vi "FRC myRIO v1.0 Read I2C.vi"(4 "Keep Bus Busy":bool, 6 "Slave Address (7-bit)":u8, 7 "Timeout ms (5)":i32=5, 8 "Error In (No Error)":errorcluster, 9 "Bytes to Read":u32) -> (0 "error out":errorcluster, 2 "Data Read":u8[](array[numeric]))   [LabVIEW 2017]
uses:
  <vilib>/rvi/errors/niLvFpgaAdjustHostInterfaceError.vi
  <vilib>/Rock Robotics/SystemInterfaces/System/FPGA_SystemFRC FPGA Ref.ctl
  <vilib>/rvi/interface/nirviReadWriteControl/nirviReadWriteControl.xnode
  NiFpgaLv.dll
  <vilib>/rvi/interface/Simulation/niFpgaSimulationCallBeginRW.vi
panel:
  # "This VI writes an array of data to the SPI Data Out register (SPIn.SPDO) and reads an array of data from the SPI Data In register (SPIn.SPDI) for a particular SPI channel (n). The data is written/read one value at a time. Please see Block Diagram for details."
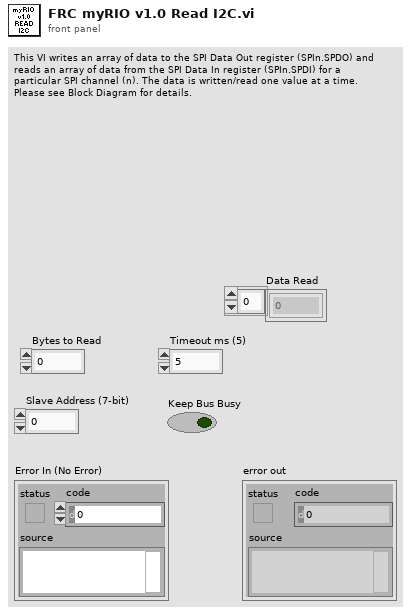
[diagram p1: front panel]
types:
  T1 = typedef "FPGA_SystemFRC FPGA Ref.ctl" = refnum<k20>
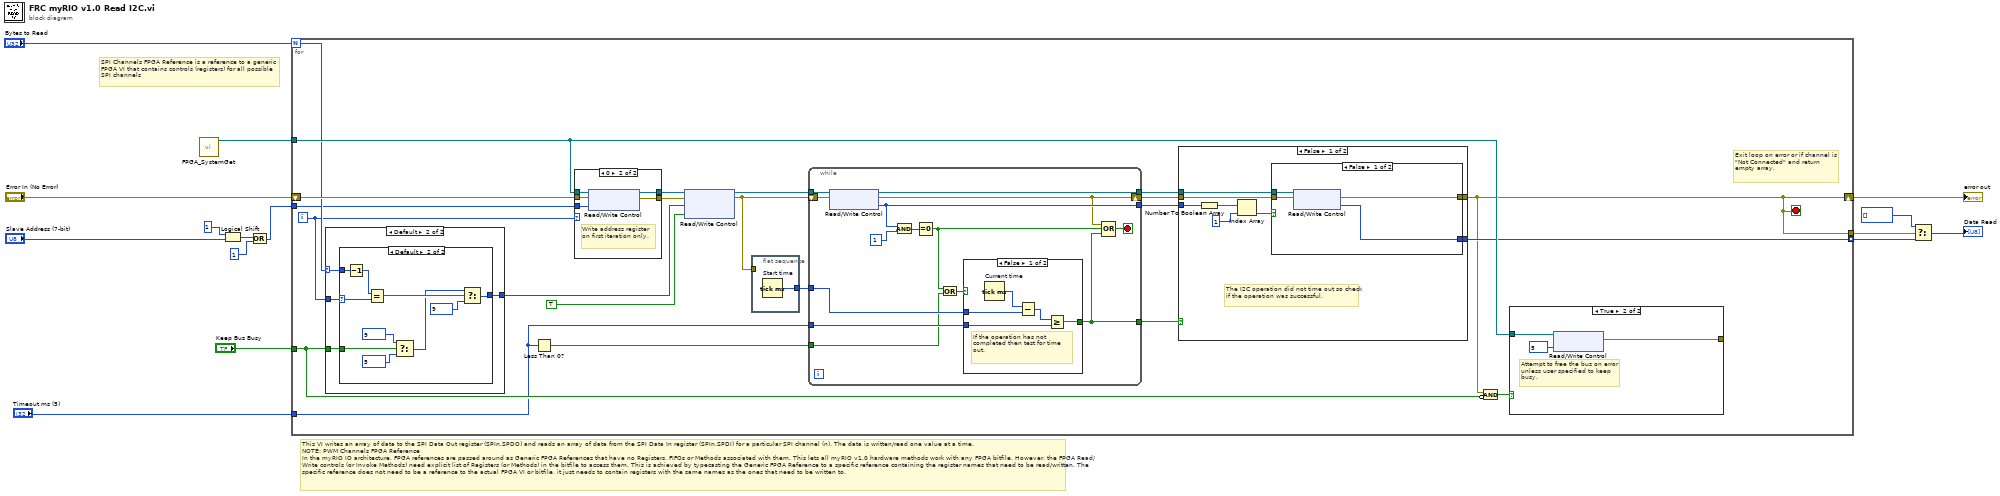
[diagram p0: block diagram]
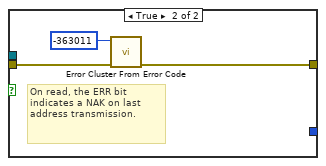
[diagram p2: hidden frame]
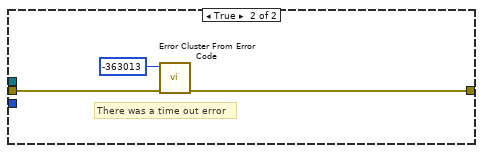
[diagram p3: hidden frame]
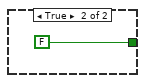
[diagram p6: hidden frame]
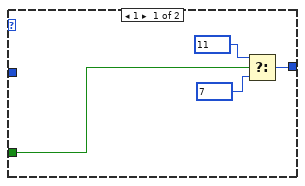
[diagram p7: hidden frame]
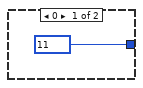
[diagram p8: hidden frame]
diagram:
  # "This VI writes an array of data to the SPI Data Out register (SPIn.SPDO) and reads an array of data from the SPI Data In register (SPIn.SPDI) for a particular SPI channel (n). The data is written/read one value at a time.\nNOTE: PWM Channels FPGA Reference\nIn the myRIO IO architecture, FPGA references are passed around as Generic FPGA References that have no Registers, FIFOs or Methods associated with them. This lets all myRIO v1.0 hardware methods work with any FPGA bitfile. However, the FPGA Read/Write controls (or Invoke Methods) need explicit list of Registers (or Methods) in the bitfile to access them. This is achieved by typecasting the Generic FPGA Reference to a specific reference containing the register names that need to be read/written. The specific reference does not need to be a reference to the actual FPGA VI or bitfile, it just needs to contain registers with the same names as the ones that need to be written to."
  # "SPI Channels FPGA Reference is a reference to a generic FPGA VI that contains controls (registers) for all possible SPI channels"
  n1 = call <vilib>:"FPGA_SystemGet.vi"() -> ("FRC FPGA Ref"=w1:T1)  [unwired: 11 in]
  n2 = Logical Shift(y=i8 1, x="Slave Address (7-bit)") -> (x << y=w13:u8)
  n3 = Or(x=w13, y=u8 1) -> (x .or. y?=w3:u8)
  n4 = for {
    N: "Bytes to Read" -> [w33]
    shift-right: [w16] -> w7
    shift-left: "Error In (No Error)" -> [w37]
    tunnel: w1 -> [w36]
    tunnel: [w32] -> w5 mode=indexing
    tunnel: [w16] -> w6
    tunnel: "Keep Bus Busy" -> [w29]
    tunnel: w3 -> [w31]
    tunnel: "Timeout ms (5)" -> [w28]
    i -> [w30]
    stop <- w16 stop-if-true
    # "Exit loop on error or if channel is \"Not Connected\" and return empty array."
    n5 = case shown="Default" w33 {
      selector: w33 -> [_ w92]
      tunnel: [w90 w93] -> w34
      tunnel: w30 -> [_ w94]
      tunnel: w29 -> [w88 w91]
      frame 1 {
        n6 = Select(t=u8 11 ("y"), s=w88, f=u8 7 ("y")) -> (s? t:f=w90:u8)
      }
      frame Default {
        n7 = case shown="Default" w94 {
          selector: w94 -> [_ w103]
          tunnel: [u8 11 ("y") w101] -> w93
          tunnel: w92 -> [_ w105]
          tunnel: w91 -> [_ w98]
          frame 0 {
          }
          frame Default {
            n8 = Decrement(x=w105) -> (x-1=w104:i32)
            n9 = Equal?(x=w104, y=w103) -> (x = y?=w102:bool)
            n10 = Select(t=u8 9 ("y"), s=w98, f=u8 5 ("y")) -> (s? t:f=w97:u8)
            n11 = Select(t=w97, s=w102, f=u8 9 ("y")) -> (s? t:f=w101:u8)
          }
        }
      }
    }
    n12 = Less Than 0?(x=w28) -> (x < 0?=w27:bool)
    n13 = case shown="0" w30 {
      tunnel: [w61 w66] -> w22
      tunnel: [w60 w65] -> w21
      tunnel: w36 -> [w61 w64]
      tunnel: w37 -> [w60 w63]
      tunnel: w31 -> [_ w62]
      frame Default {
      }
      frame 0 {
        # "Write address register on first iteration only."
        n14 = xnode "Read/Write Control"("FPGA VI Reference In"=w64, "error in"=w63, "Accel.ADDR"=w62) -> ("FPGA VI Reference Out"=w66:T1, "error out"=w65:errorcluster)
      }
    }
    n15 = xnode "Read/Write Control"("FPGA VI Reference In"=w22, "error in"=w21, "Accel.CNTL"=w34, "Accel.GO"=TRUE ("I2C0.GO")) -> ("FPGA VI Reference Out"=w26:T1, "error out"=w17:errorcluster)
    n16 = flat-sequence {
      tunnel: [w38] -> w19
      tunnel: w17 -> [_]
      frame #0 {
        n17 = Tick Count (ms) "Start time"() -> (millisecond timer value=w38:u32)
      }
    }
    n18 = while {
      tunnel: w26 -> [w79]
      shift-right: [w73] -> w25
      shift-left: w17 -> [w80]
      tunnel: [w75] -> w24
      tunnel: [w74] -> w23
      tunnel: w19 -> [w72]
      tunnel: [w71] -> w18
      tunnel: w28 -> [w70]
      tunnel: w27 -> [w68]
      stop <- w76 stop-if-true
      n19 = xnode "Read/Write Control"("FPGA VI Reference In"=w79, "error in"=w80) -> ("FPGA VI Reference Out"=w74:T1, "error out"=w73:errorcluster, "Accel.STAT"=w75:u8)
      n20 = And(x=w75, y=u8 1) -> (x .and. y?=w77:u8)
      n21 = Equal To 0?(x=w77) -> (x = 0?=w67:bool)
      n22 = Or(x=w67, y=w68) -> (x .or. y?=w69:bool)
      n23 = case shown="False" w69 {
        tunnel: w72 -> [w83 _]
        tunnel: [w82 FALSE] -> w71
        tunnel: w70 -> [w81 _]
        frame False {
          # "If the operation has not completed then test for time out."
          n24 = Tick Count (ms) "Current time"() -> (millisecond timer value=w84:u32)
          n25 = Subtract(x=w84, y=w83) -> (x-y=w85:u32)
          n26 = Greater Or Equal?(x=w85, y=w81) -> (x >= y?=w82:bool)
        }
        frame True {
        }
      }
      n27 = Compound Arithmetic op=OR(w73, w67, w71) -> (w76:bool)
    }
    n28 = case shown="False" w18 {
      tunnel: w25 -> [w46 w55]
      tunnel: w24 -> [w45 _]
      tunnel: [w41 _] -> w32
      tunnel: w23 -> [w40 _]
      tunnel: [w39 w54] -> w16
      frame False {
        # "The I2C operation did not time out so check if the operation was successful."
        n29 = Number To Boolean Array(number=w45) -> (Boolean array=w44:bool[])
        n30 = Index Array(array=w44, index=1) -> (element=w43:bool)
        n31 = case shown="False" w43 {
          tunnel: w46 -> [w48 w51]
          tunnel: [w49 w53] -> w39
          tunnel: [w50 _] -> w41
          tunnel: w40 -> [w47 _]
          frame False {
            n32 = xnode "Read/Write Control"("FPGA VI Reference In"=w47, "error in"=w48) -> ("error out"=w49:errorcluster, "Accel.DATI"=w50:u8)  [unwired: 1 out]
          }
          frame True {
            # "On read, the ERR bit indicates a NAK on last address transmission."
            n33 = call <vilib>:"Error Cluster From Error Code.vi"("error in (no error)"=w51, "error code (0)"=-363011) -> ("error out"=w53:errorcluster)  [unwired: 7 in]
          }
        }
      }
      frame True {
        # "There was a time out error"
        n34 = call <vilib>:"Error Cluster From Error Code.vi"("error in (no error)"=w55, "error code (0)"=-363013) -> ("error out"=w54:errorcluster)  [unwired: 7 in]
      }
    }
    n35 = Compound Arithmetic op=AND(w16, invert w29) -> (w20:bool)
    n36 = case shown="True" w20 {
      tunnel: w36 -> [_ w59]
      tunnel: [_ w57] -> _
      frame False {
      }
      frame True {
        # "Attempt to free the bus on error unless user specified to keep busy."
        n37 = xnode "Read/Write Control"("FPGA VI Reference In"=w59, "Accel.CNTL"=u8 5 ("I2C.C_0.CNTL")) -> ("error out"=w57:errorcluster)  [unwired: 1 in, 1 out]
      }
    }
  }
  "error out" <- w7
  n38 = Select(t=u8[] [], s=w6, f=w5) -> (s? t:f=→"Data Read":u8[])
